vi "log save.vi"(11 "Instrument":T4={"335 Resource"="GPIB0::24::INSTR", "Input (0:A)"=0, "Instrument Type"=enum."SVSM", "quantum design"=refnum, "Heater Output (1:1)"=1, "semaphore"=refnum, "TCP master instance"=refnum, "335 Status"=refnum, "M24C Resource"="GPIB0::24::INSTR", "4G supply"="GPIB0::24::INSTR", "Temp Status 24C"=refnum, "Temp"=refnum, "9T信号"=refnum, "4g supply status"=refnum, "limit"={"Field limit"=0.0, "Field rate limit"=0.0, "Temp limit"=0.0, "Temp low limit"=0.0, "Temp rate limit "=0.0}} {"Input (0:A)" items=["A", "B"]; "Heater Output (1:1)" items=["1"=1, "2"=2]}) -> ()   [LabVIEW 2019, in "SubVI.lvlib"]
uses:
  SubVI.lvlib
  Instrument.ctl
  <vilib>/NI/Modbus Library/API/Master/Modbus Master.lvclass
  Instrument Type.ctl
  lib/QDInstrument.dll
  335 state.ctl
  9T mag field stauts.ctl
  limit.ctl
  <vilib>/Utility/file.llb/Write Delimited Spreadsheet (string).vi
  9T cmag.lvlib
panel:
  out "field stauts":T1=enum."Stable"
  in  "枚举":T2(ring)
  out "Temp Status":T3 items=["Unknow", "Stable", "Following Warm", "Following Cold", "Unfollowing"]
  out "Temperature\nStatus 2":i32(ring) items=["TemperatureUnknown"=0, "Stable"=1, "Tracking"=2, "Near"=5, "Chasing"=6, "Filling"=7, "Standby"=10, "Disabled"=13, "ImpedanceNotFunction"=14, "TempFailure"=15]
  out "Chamber\nStatus 2":i32(ring) items=["ChamberUnknown"=0, "PurgedAndSealed"=1, "VentedAndSealed"=2, "Sealed"=3, "Purging"=4, "Venting"=5, "PreHiVac"=6, "HighVac"=7, "PumpContinuous"=8, "VentContinuous"=9, "ChamberFailure"=15]
  out "Field\nStatus 2":i32(ring) items=["MagnetUnknown"=0, "StablePersistent"=1, "WarmingSwitch"=2, "CoolingSwitch"=3, "StableDriven"=4, "Iterating"=5, "Charging"=6, "Discharging"=7, "CurrentError"=8, "MagnetFailure"=15]
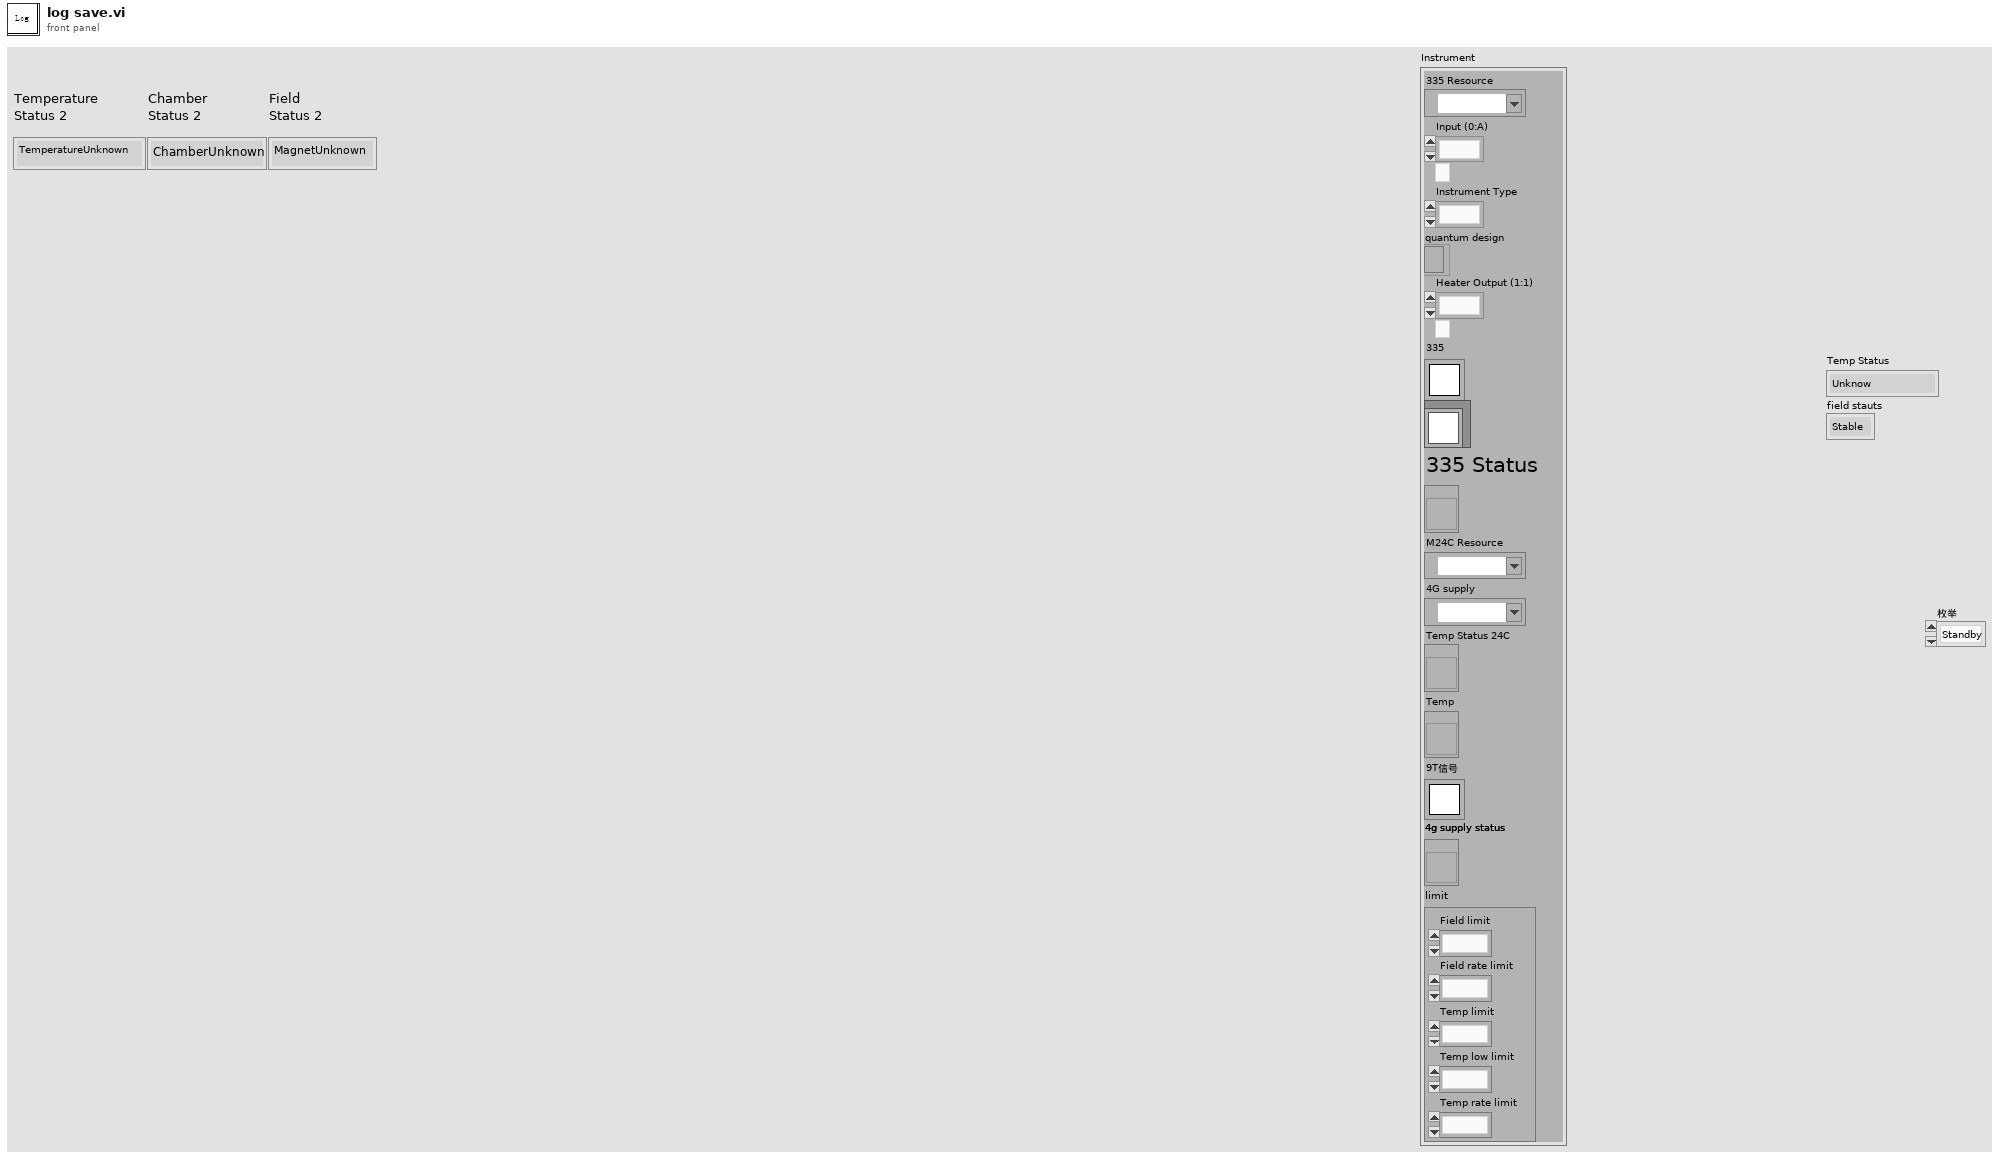
[diagram p1: front panel]
types:
  T1 = typedef "9T mag field stauts.ctl" = enum16{"unknow", "Stable", "Sweep up", "Sweep down", "Sweep to zero"}
  T2 = enum16{"Standby", "sweep up ", "sweep down", "sweep paused", "zeroing", "sweep up fast", "sweep down ", "zeroing fast"}
  T3 = typedef "335 state.ctl" = u16
  T4 = typedef "Instrument.ctl" = cluster{"335 Resource":refnum<visa-resource-name>, "Input (0:A)":u16, "Instrument Type":T5, "quantum design":refnum<k24>, "Heater Output (1:1)":u16, "semaphore":T6, "TCP master instance":refnum<class "Modbus Master.lvclass">, "335 Status":refnum<vi>, "M24C Resource":refnum<visa-resource-name>, "4G supply":refnum<visa-resource-name>, "Temp Status 24C":refnum<vi>, "Temp":refnum<vi>, "9T信号":T6, "4g supply status":refnum<vi>, "limit":T7}
  T5 = typedef "Instrument Type.ctl" = enum16{"PPMS", "VersaLab", "DynaCool", "SVSM", "PPMS-Rotate", "Lakeshore335", "9T mag"}
  T6 = typedef "Semaphore RefNum" = refnum<k1>
  T7 = typedef "limit.ctl" = cluster{"Field limit":dbl, "Field rate limit":dbl, "Temp limit":dbl, "Temp low limit":dbl, "Temp rate limit ":dbl}
  T8 = enum16{"open", "replace", "create", "open or create", "replace or create", "replace or create with confirmation"}
  T9 = cluster{"Temperature A":dbl, "Temperature B":dbl, "Temperature C":dbl, "Temperature D":dbl, "Loop1 Ramp?":bool, "Loop2 Ramp?":bool, "Loop1 Setpoint":dbl, "Loop2 Setpoint":dbl, "Output Pwr (%)":dbl, "Output Pwr (%)":dbl}
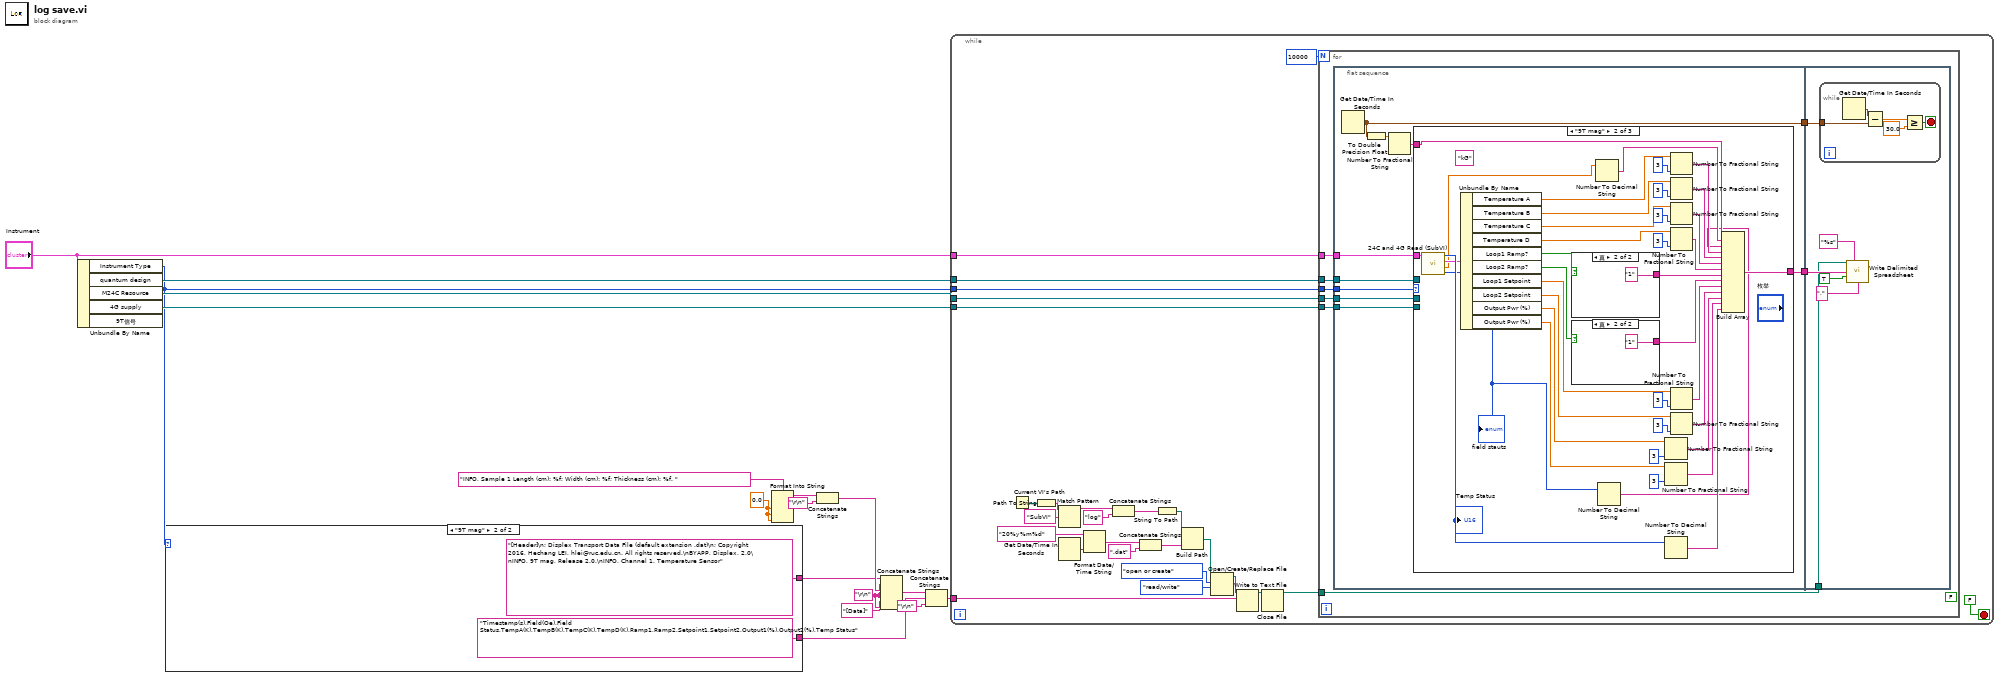
[diagram p0: block diagram]
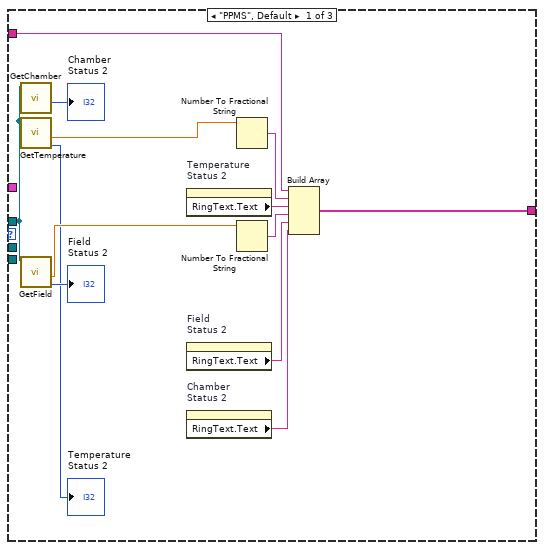
[diagram p2: hidden frame]
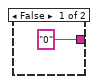
[diagram p3: hidden frame]
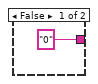
[diagram p4: hidden frame]
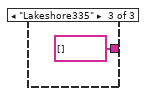
[diagram p5: hidden frame]
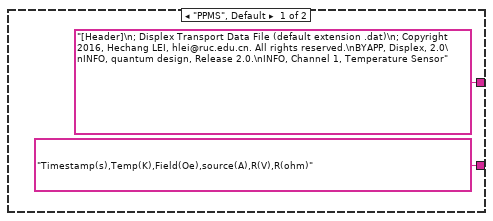
[diagram p6: hidden frame]
diagram:
  w7 = 0.0 ("输入 1")
  w4 = "\r\n"
  n1 = Unbundle By Name("Instrument") -> ("Instrument Type"=w13:T5, "quantum design"=w17:refnum<k24>, "M24C Resource"=w16:refnum<visa-resource-name>, "4G supply"=w15:refnum<visa-resource-name>)  [unwired: 1 out]
  n2 = case shown="\"9T mag\"" w13 {
    tunnel: ["[Header]\n; Displex Transport Data File (default extension .dat)\n; Copyright 2016, Hechang LEI, hlei@ruc.edu.cn. All rights reserved.\nBYAPP, Displex, 2.0\nINFO, quantum design, Release 2.0.\nINFO, Channel 1, Temperature Sensor" ("string") "[Header]\n; Displex Transport Data File (default extension .dat)\n; Copyright 2016, Hechang LEI, hlei@ruc.edu.cn. All rights reserved.\nBYAPP, Displex, 2.0\nINFO, 9T mag, Release 2.0.\nINFO, Channel 1, Temperature Sensor" ("string")] -> w5
    tunnel: ["Timestamp(s),Temp(K),Field(Oe),source(A),R(V),R(ohm)" ("字符串") "Timestamp(s),Field(Oe),Field Status,TempA(K),TempB(K),TempC(K),TempD(K),Ramp1,Ramp2,Setpoint1,Setpoint2,Output1(%),Output2(%),Temp Status" ("字符串")] -> w1
    frame "PPMS", Default {
    }
    frame "9T mag" {
    }
  }
  n3 = Format Into String(format string="INFO, Sample 1 Length (cm): %f; Width (cm): %f; Thickness (cm): %f. " ("string"), w7, w7, w7) -> (resulting string=w11:string)  [unwired: 2 in, 1 out]
  n4 = Concatenate Strings(w11, "\r\n") -> (w9:string)
  n5 = Concatenate Strings(w5, w4, w9, w4, "[Data]" ("string"), w4) -> (w10:string)
  n6 = Concatenate Strings(w10, w1, "\r\n") -> (w12:string)
  n7 = while {
    tunnel: w17 -> [w47]
    tunnel: w16 -> [w46]
    tunnel: w15 -> [w45]
    tunnel: "Instrument" -> [w44]
    tunnel: w13 -> [w43]
    tunnel: w12 -> [w40]
    stop <- FALSE stop-if-true
    n8 = Current VI's Path() -> (path=w36:path)
    n9 = Path To String(path=w36) -> (string=w35:string)
    n10 = Match Pattern(string=w35, regular expression="SubVI" ("正则表达式")) -> (before substring=w33:string)  [unwired: 1 in, 3 out]
    n11 = Get Date/Time In Seconds() -> (seconds since 1Jan1904=w28:timestamp)
    n12 = Format Date/Time String(time format string (%c)="20%y%m%d" ("时间格式字符串(%c)"), seconds (now)=w28) -> (date/time string=w26:string)  [unwired: 1 in]
    n13 = Concatenate Strings(w33, "log" ("字符串")) -> (w31:string)
    n14 = Concatenate Strings(w26, ".dat" ("字符串")) -> (w25:string)
    n15 = String To Path(string=w31) -> (path=w30:path)
    n16 = Build Path(base path=w30, name or relative path=w25) -> (appended path=w24:path)
    n17 = Open/Create/Replace File(file path (use dialog)=w24, operation (0:open)=T8."open or create" ("操作(0:open)"), access (0:read/write)=enum16{"read/write", "read-only", "write-only"}."read/write" ("权限(0:read/write)")) -> (refnum out=w41:refnum<file>)  [unwired: 3 in, 2 out]
    n18 = Write to Text File(file (use dialog)=w41, text=w40) -> (refnum out=w42:refnum<file>)  [unwired: 2 in, 2 out]
    n19 = Close File(refnum=w42) -> (path=w37:path)  [unwired: 1 in, 1 out]
    n20 = for {
      N: 10000 -> [_]
      tunnel: w47 -> [w55]
      tunnel: w43 -> [w52]
      tunnel: w46 -> [w51]
      tunnel: w45 -> [w50]
      tunnel: w44 -> [w49]
      tunnel: w37 -> [w48]
      (unwired) FALSE
      n21 = flat-sequence {
        tunnel: w55 -> [w64]
        tunnel: [w62] -> w54
        tunnel: [w63] -> w53
        tunnel: w52 -> [w61]
        tunnel: w51 -> [w60]
        tunnel: w50 -> [w59]
        tunnel: w49 -> [w58]
        tunnel: w54 -> [w123]
        tunnel: w53 -> [w122]
        tunnel: w48 -> [w121]
        frame #0 {
          n22 = Get Date/Time In Seconds() -> (seconds since 1Jan1904=w62:timestamp)
          n23 = To Double Precision Float(number=w62) -> (double precision float=w56:dbl)
          n24 = Number To Fractional String(number=w56) -> (F-format string=w57:string)  [unwired: 3 in]
          n25 = case shown="\"9T mag\"" w61 {
            tunnel: w64 -> [w77 _ _]
            tunnel: [w66 w86 string[] []] -> w63
            tunnel: w60 -> [_ _ _]
            tunnel: w59 -> [_ _ _]
            tunnel: w58 -> [_ w115 _]
            tunnel: w57 -> [w65 w84 _]
            frame "PPMS", Default {
              n26 = call "GetChamber.vi"("Instrument Ref In"=w77) -> ("Chamber\nStatus"=→"Chamber\nStatus 2":i32)  [unwired: 3 in, 3 out]
              n27 = call "GetTemperature.vi"("Instrument Ref In"=w77) -> ("Temperature\nStatus"=→"Temperature\nStatus 2":i32, "Temperature"=w71:dbl)  [unwired: 4 in, 3 out]
              n28 = call "GetField.vi"("Instrument Ref In"=w77) -> ("Field\nStatus"=→"Field\nStatus 2":i32, "Field"=w70:dbl)  [unwired: 4 in, 3 out]
              n29 = property on="Temperature\nStatus 2" class="Ring (严格)"() -> ("RingText.Text"=w73:string)  [unwired: 2 in, 2 out]
              n30 = property on="Field\nStatus 2" class="Ring (严格)"() -> ("RingText.Text"=w75:string)  [unwired: 2 in, 2 out]
              n31 = property on="Chamber\nStatus 2" class="Ring (严格)"() -> ("RingText.Text"=w76:string)  [unwired: 2 in, 2 out]
              n32 = Number To Fractional String(number=w71) -> (F-format string=w72:string)  [unwired: 3 in]
              n33 = Number To Fractional String(number=w70) -> (F-format string=w74:string)  [unwired: 3 in]
              n34 = Build Array(w65, w72, w73, w74, w75, w76) -> (w66:string[])
            }
            frame "9T mag" {
              (unwired) "kG" ("正则表达式")
              n35 = call "24C and 4G Read (SubVI).vi"("Instrument"=w115) -> ("field status"=w79:T1, "field(Oe)"=w81:dbl, "输出簇"=w113:T9, "下拉列表"=w114:T3)  [unwired: 7 in]
              "Temp Status" <- w114
              "field stauts" <- w79
              n36 = Unbundle By Name(w113) -> ("Temperature A"=w104:dbl, "Temperature B"=w103:dbl, "Temperature C"=w102:dbl, "Temperature D"=w101:dbl, "Loop1 Ramp?"=w95:bool, "Loop2 Ramp?"=w96:bool, "Loop1 Setpoint"=w92:dbl, "Loop2 Setpoint"=w89:dbl, "Output Pwr (%)"=w106:dbl, "Output Pwr (%)"=w105:dbl)
              n37 = case shown="真" w95 {
                tunnel: ["0" "1"] -> w94
                frame False {
                }
                frame True {
                }
              }
              n38 = case shown="真" w96 {
                tunnel: ["0" "1"] -> w93
                frame False {
                }
                frame True {
                }
              }
              n39 = Number To Decimal String(number=w81) -> (decimal integer string=w80:string)  [unwired: 1 in]
              n40 = Number To Decimal String(number=w79) -> (decimal integer string=w78:string)  [unwired: 1 in]
              n41 = Number To Fractional String(number=w106, precision (6)=i16 3) -> (F-format string=w88:string)  [unwired: 2 in]
              n42 = Number To Fractional String(number=w105, precision (6)=i16 3) -> (F-format string=w87:string)  [unwired: 2 in]
              n43 = Number To Decimal String(number=w114) -> (decimal integer string=w85:string)  [unwired: 1 in]
              n44 = Number To Fractional String(number=w104, precision (6)=i16 3 ("精度(6)")) -> (F-format string=w100:string)  [unwired: 2 in]
              n45 = Number To Fractional String(number=w103, precision (6)=i16 3 ("精度(6)")) -> (F-format string=w99:string)  [unwired: 2 in]
              n46 = Number To Fractional String(number=w102, precision (6)=i16 3 ("精度(6)")) -> (F-format string=w98:string)  [unwired: 2 in]
              n47 = Number To Fractional String(number=w101, precision (6)=i16 3 ("精度(6)")) -> (F-format string=w97:string)  [unwired: 2 in]
              n48 = Number To Fractional String(number=w92, precision (6)=i16 3 ("精度(6)")) -> (F-format string=w91:string)  [unwired: 2 in]
              n49 = Number To Fractional String(number=w89, precision (6)=i16 3 ("精度(6)")) -> (F-format string=w90:string)  [unwired: 2 in]
              n50 = Build Array(w84, w80, w78, w100, w99, w98, w97, w94, w93, w91, w90, w88, w87, w85) -> (w86:string[])
            }
            frame "Lakeshore335" {
            }
          }
        }
        frame #1 {
          n51 = while {
            tunnel: w123 -> [w130]
            stop <- w128 stop-if-true
            n52 = Get Date/Time In Seconds() -> (seconds since 1Jan1904=w131:timestamp)
            n53 = Subtract(x=w131, y=w130) -> (x-y=w129:dbl)
            n54 = Greater Or Equal?(x=w129, y=30.0 ("log.log interval")) -> (x >= y?=w128:bool)
          }
          n55 = call-poly <vilib>:"Write Delimited Spreadsheet.vi"("file path (dialog if empty)"=w121, "format (%s)"="%s", "1D data"=w122, "append to file? (new file:F)"=TRUE, "delimiter (\\t)"="," ("delimiter (\\t)")) -> ()  [unwired: 9 in, 2 out]
        }
      }
    }
  }
